vi "Add Project Item.vi"(8 "error in (no error)":errorcluster, 10 "Folder Location Ref":refnum<vi>, 11 "IO Class in":refnum<class "Signal.lvclass">) -> (0 "error out":errorcluster, 3 "IO Class out":refnum<class "Signal.lvclass">)   [LabVIEW 2015, in "Signal.lvclass"]
uses:
  Signal.lvclass
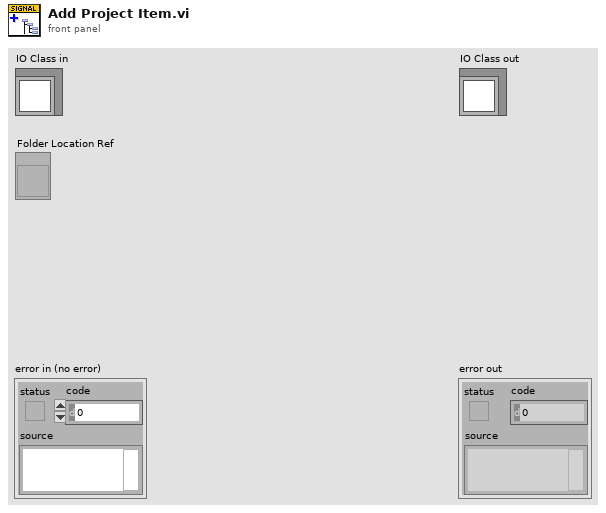
[diagram p1: front panel]
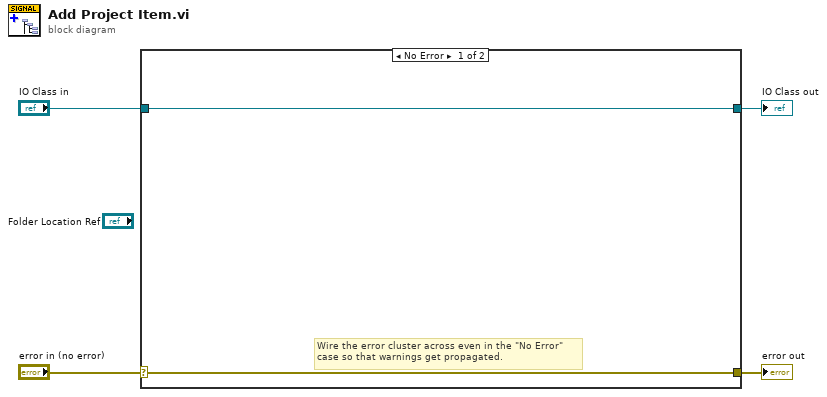
[diagram p0: block diagram]
diagram:
  n1 = case shown="No Error" "error in (no error)" {
    selector: "error in (no error)" -> [w5 w8]
    tunnel: [w5 w8] -> w3
    tunnel: [w6 w7] -> w1
    tunnel: "IO Class in" -> [w6 w7]
    frame No Error {
      # "Wire the error cluster across even in the \"No Error\"\ncase so that warnings get propagated."
    }
    frame Error {
    }
  }
  "error out" <- w3
  "IO Class out" <- w1
